vi "FeedbackDecode_SendMSMSPacket.vi"(1 "CompArrayIn":T1(array[cluster]), 3 "CompVal":sgl[][](array[numeric]), 4 "FNum":i16[](array[numeric]), 5 "CompIdx":i32[](array[numeric]), 6 "Mode":enum16{"Initialize", "Run", "Close"}(ring)) -> ()   [LabVIEW 2020]
panel:
  out "CompArray":T1(array[cluster])
  out "UDPID":refnum<k16>
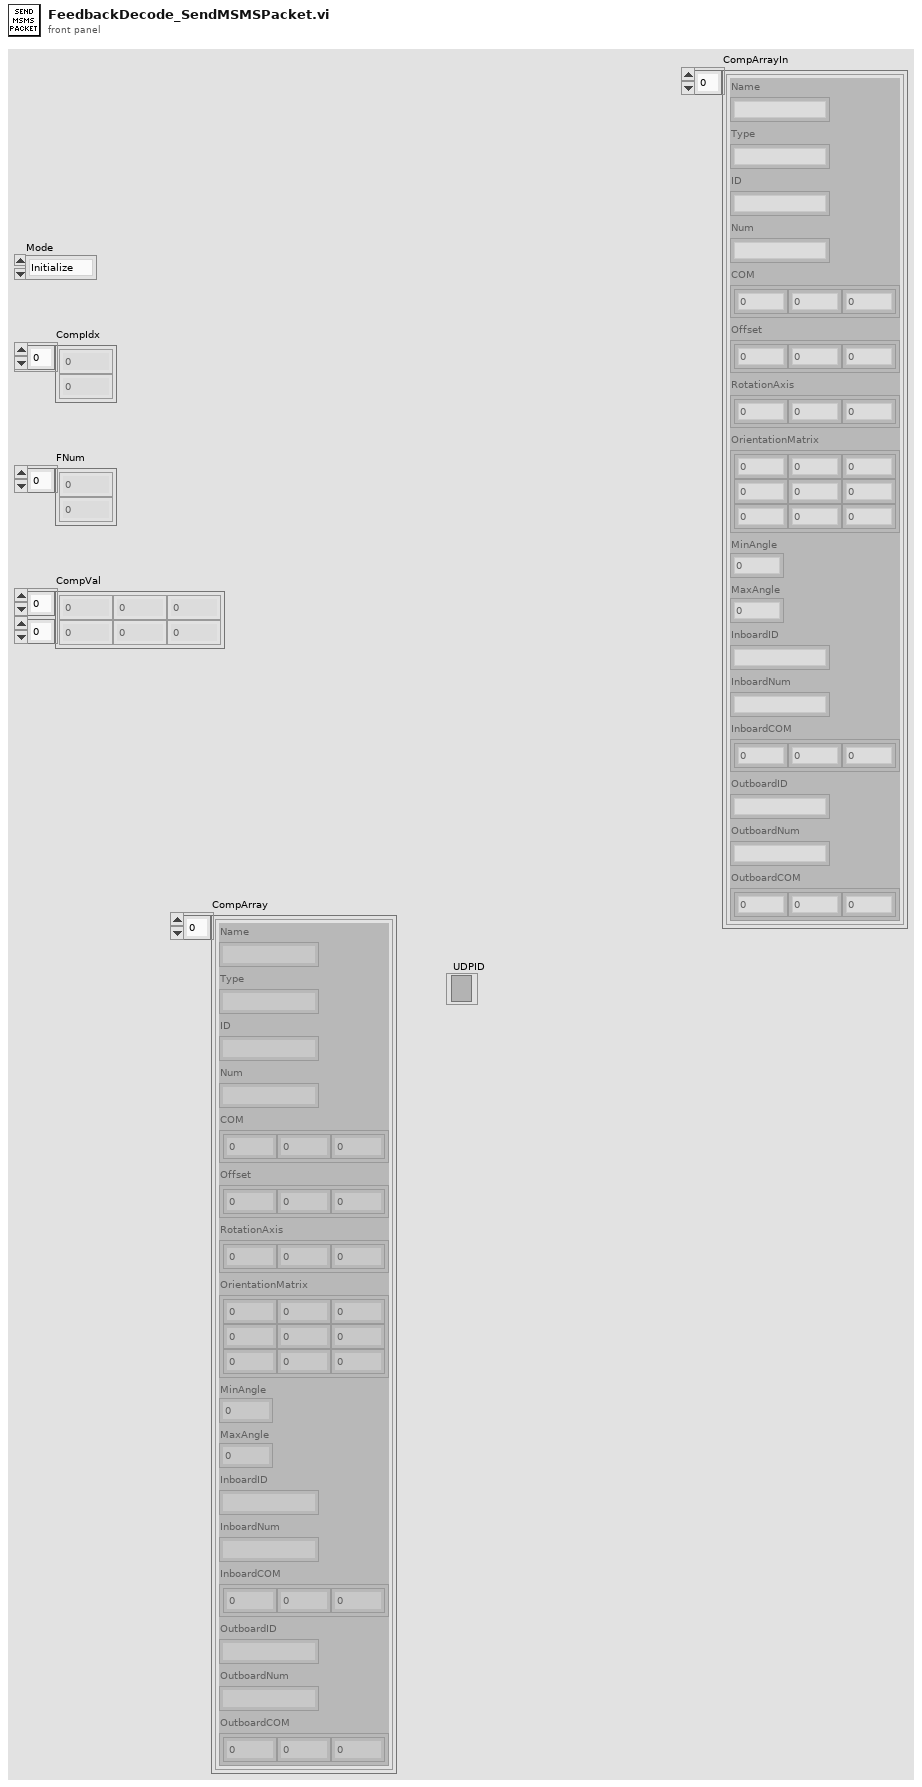
[diagram p1: front panel]
types:
  T1 = cluster{"Name":string, "Type":string, "ID":string, "Num":string, "COM":dbl[], "Offset":dbl[], "RotationAxis":dbl[], "OrientationMatrix":dbl[][], "MinAngle":dbl, "MaxAngle":dbl, "InboardID":string, "InboardNum":string, "InboardCOM":dbl[], "OutboardID":string, "OutboardNum":string, "OutboardCOM":dbl[]}[]
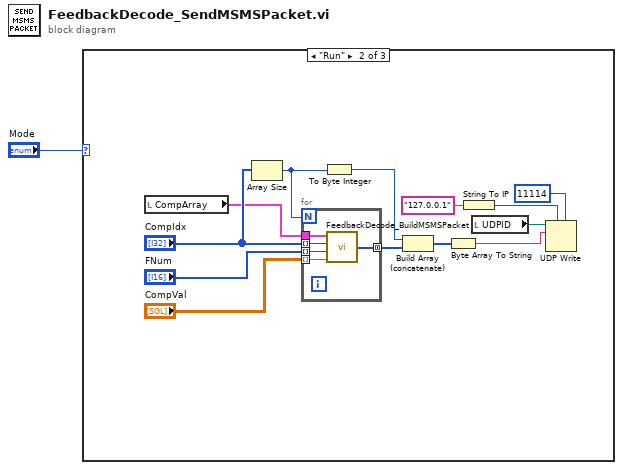
[diagram p0: block diagram]
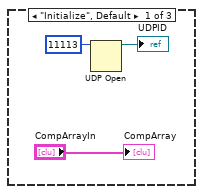
[diagram p2: hidden frame]
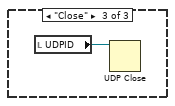
[diagram p3: hidden frame]
diagram:
  n1 = case shown="\"Run\"" "Mode" {
    frame "Initialize", Default {
      n2 = UDP Open(11:u16 11113 ("port")) -> (port=→"UDPID":refnum<k16>)  [unwired: 4 in, 2 out]
      "CompArray" <- "CompArrayIn"
    }
    frame "Run" {
      n3 = local read "CompArray"() -> (w5:T1)
      n4 = Array Size(array="CompIdx") -> (size(s)=w16:i32)
      n5 = for {
        N: w16 -> [_]
        tunnel: "CompIdx" -> [w22] mode=indexing
        tunnel: "FNum" -> [w21] mode=indexing
        tunnel: "CompVal" -> [w20] mode=indexing
        tunnel: [w19] -> w13 mode=concatenating
        tunnel: w5 -> [w18]
        n6 = call "FeedbackDecode_BuildMSMSPacket.vi"("Value"=w20, "FNum"=w21, "CompIdx"=w22, "CompArray"=w18) -> ("CompPacket"=w19:i8[])
      }
      n7 = To Byte Integer(number=w16) -> (8bit integer=w15:i8)
      n8 = Build Array (concatenate)(w15, w13) -> (w10:i8[])
      n9 = Byte Array To String(unsigned byte array=w10) -> (string=w9:string)
      n10 = String To IP(1:"127.0.0.1" ("name")) -> (0:w8:u32)
      n11 = local read "UDPID"() -> (w17:refnum<k16>)
      n12 = UDP Write(address=w8, port or service name=u16 11114 ("port"), connection ID=w17, data in=w9) -> ()  [unwired: 2 in, 2 out]
    }
    frame "Close" {
      n13 = local read "UDPID"() -> (w23:refnum<k16>)
      n14 = UDP Close(connection ID=w23) -> ()  [unwired: 1 in, 2 out]
    }
  }
